vi "Write Conversion Time.vi"(8 "error in":errorcluster, 10 "conversion time":T1, 11 "NI 9228 in":refnum<class "NI 9228.lvclass">) -> (0 "error out":errorcluster, 3 "NI 9228 out":refnum<class "NI 9228.lvclass">)   [LabVIEW 2019, in "Scan Engine Scripting.lvlib" / "NI 9228.lvclass"]
uses:
  NI 9228.lvclass
  Utility/Shared Properties/Conversion Time.ctl
  NI 9228.lvclass/NI 9228.ctl
  Scan Engine Scripting.lvlib
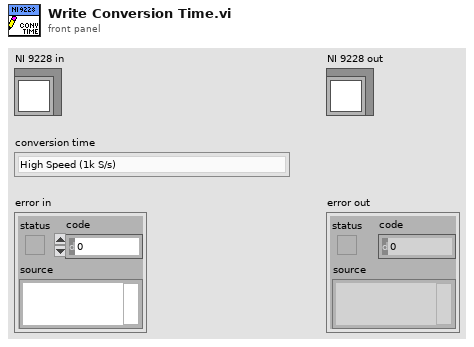
[diagram p1: front panel]
types:
  T1 = typedef "Scan Engine Scripting.lvlib/Conversion Time.ctl" = enum16{"High Speed (1k S/s)", "Medium Speed (100 S/s)", "Medium Resolution (50/60Hz Rejection - 12 S/s)", "High Resolution (50/60Hz Rejection - 2 S/s)"}
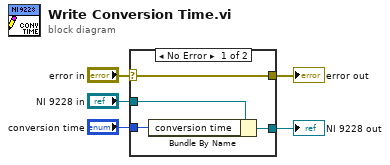
[diagram p0: block diagram]
diagram:
  n1 = case shown="No Error" "error in" {
    selector: "error in" -> [w9 w10]
    tunnel: [w9 w10] -> w4
    tunnel: [w7 w11] -> w2
    tunnel: "NI 9228 in" -> [w8 w11]
    tunnel: "conversion time" -> [w6 _]
    frame No Error {
      n2 = Bundle By Name(cluster=w8, "conversion time"=w6) -> (w7:refnum<class "NI 9228.lvclass">)
    }
    frame Error {
    }
  }
  "error out" <- w4
  "NI 9228 out" <- w2
